vi "Ctor.vi"(8 "error in (no error)":errorcluster, 11 "Value":string) -> (0 "error out":errorcluster, 3 "Test Type A out":refnum<class "Test Type A.lvclass">)   [LabVIEW 2020, in "Test Type A.lvclass"]
uses:
  Test Type A.lvclass
  Ref Data.ctl
  Test Type A.lvclass/Test Type A.ctl
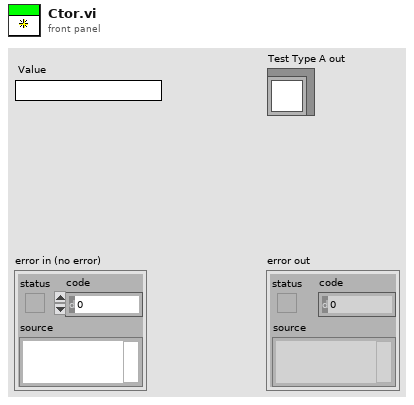
[diagram p1: front panel]
types:
  T1 = typedef "Test Type A.lvclass/Ref Data.ctl" = cluster{"Value":string}
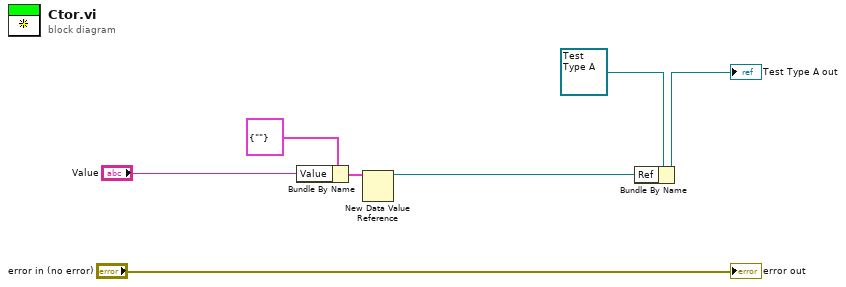
[diagram p0: block diagram]
diagram:
  n1 = Bundle By Name(cluster=T1 {"Value"=""} ("Ref Data"), "Value"="Value") -> (w3:T1)
  n2 = New Data Value Reference(data value=w3) -> (data value reference=w1:refnum<data-value>)  [unwired: 1 in, 1 out]
  n3 = Bundle By Name(cluster=refnum<class "Test Type A.lvclass"> refnum ("Test Type A in"), "Ref"=w1) -> (→"Test Type A out":refnum<class "Test Type A.lvclass">)
  "error out" <- "error in (no error)"
